vi "Spreadsheet Example.vi"() -> ()   [LabVIEW 2012]
doc: "该VI是LabVIEW核心课程1中的练习。\n\n该VI将生成3个数据数组，将其组合为二维数组并在图表中显示。通过“写入电子表格文件”高级文件I/O函数将二维数组数据写入电子表格文件。"
uses:
  <vilib>/Utility/file.llb/Write To Spreadsheet File (DBL).vi
  <vilib>/Analysis/NI_AALBase.lvlib
panel:
  out "表格":string[][](table)
  out "波形图":dbl[][](graph)
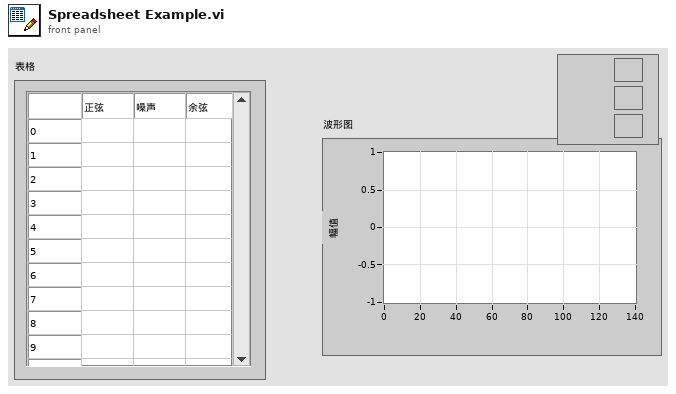
[diagram p1: front panel]
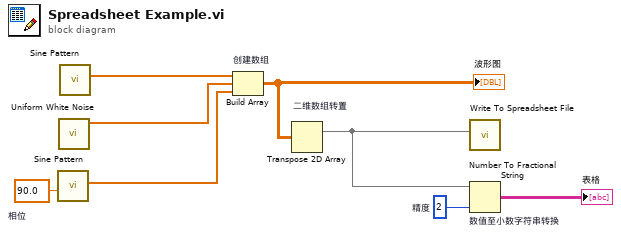
[diagram p0: block diagram]
diagram:
  w5 = 2  # 精度
  w6 = 90.0  # 相位
  n1 = call <vilib>:"Sine Pattern.vi"("phase(degrees)"=w6) -> ("Sinusoidal Pattern"=w3:dbl[])  [unwired: 3 in, 1 out]
  n2 = call <vilib>:"Uniform White Noise.vi"() -> ("uniform white noise"=w8:dbl[])  [unwired: 10 in, 1 out]
  n3 = call <vilib>:"Sine Pattern.vi"() -> ("Sinusoidal Pattern"=w7:dbl[])  [unwired: 4 in, 1 out]
  n4 = Build Array "创建数组"(w7, w8, w3) -> (w1:dbl[][])
  "波形图" <- w1
  n5 = Transpose 2D Array "二维数组转置"(2D array=w1) -> (transposed array=w4:dbl[][])
  n6 = call-poly <vilib>:"Write To Spreadsheet File.vi"("2D data"=w4) -> ()  [unwired: 7 in, 1 out]
  n7 = Number To Fractional String "数值至小数字符串转换"(number=w4, precision (6)=w5) -> (F-format string=→"表格":string[][])  [unwired: 2 in]
